vi "SingleOutPutA.vi"(8 "error in (no error)":errorcluster, 9 "Bool":bool, 10 "Index":i32, 11 "ZanCard in":refnum<class "ZanCard.lvclass">) -> (0 "error out":errorcluster, 3 "ZanCard out":refnum<class "ZanCard.lvclass">)   [LabVIEW 2019, in "ZanCard.lvclass"]
uses:
  ZanCard.lvclass
  ZanCard.lvclass/ZanCard.ctl
  LLB/zmotion/zaux/zauxdll.lvlib
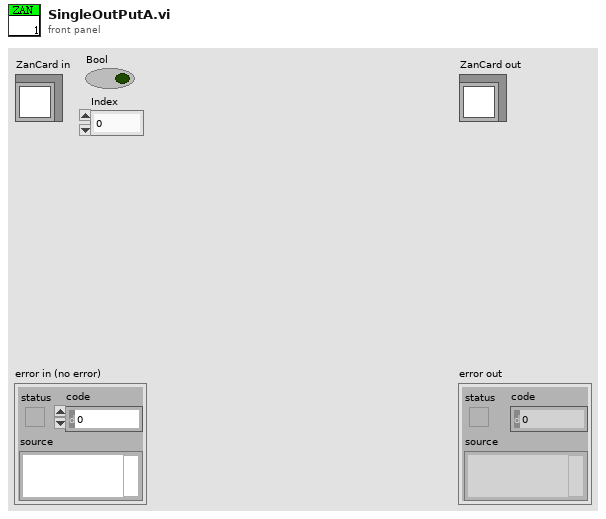
[diagram p1: front panel]
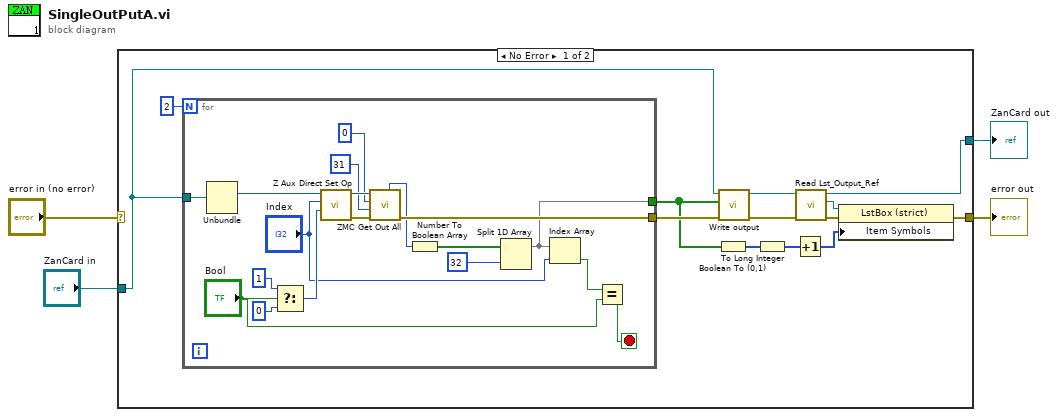
[diagram p0: block diagram]
diagram:
  n1 = case shown="No Error" "error in (no error)" {
    selector: "error in (no error)" -> [_ w37]
    tunnel: "ZanCard in" -> [w17 w36]
    tunnel: [w14 w36] -> w2
    tunnel: [w11 w37] -> w1
    frame No Error {
      n2 = for {
        N: 2 -> [_]
        tunnel: w17 -> [w31]
        tunnel: [w25] -> w10
        tunnel: [w19] -> w5
        stop <- w18 stop-if-true
        n3 = Unbundle(w31) -> (w35:i32)  [unwired: 3 out]
        n4 = Select(t=1, s="Bool", f=0) -> (s? t:f=w32:i32)
        n5 = call "Z Aux Direct Set Op.vi"("iValue"=w32, "ionum"="Index", "handle"=w35) -> ("error out"=w24:errorcluster, "handle out"=w30:u32)  [unwired: 6 in, 1 out]
        n6 = call "ZMC Get Out All.vi"("error in (no error)"=w24, "inumend"=31 ("ionumend"), "inumfirst"=0 ("ionumfirst"), "handle"=w30) -> ("error out"=w25:errorcluster, "pistate out"=w23:u32)  [unwired: 4 in, 2 out]
        n7 = Number To Boolean Array(number=w23) -> (Boolean array=w27:bool[])
        n8 = Split 1D Array(array=w27, index=32) -> (first subarray=w19:bool[])  [unwired: 1 out]
        n9 = Index Array(array=w19, index="Index") -> (element=w21:bool)
        n10 = Equal?(x=w21, y="Bool") -> (x = y?=w18:bool)
      }
      n11 = Boolean To (0,1)(Boolean=w5) -> (0, 1=w9:i16[])
      n12 = call-dynamic "Write output.vi"("error in (no error)"=w10, "output"=w5, "IOCard in"=w17) -> ("error out"=w13:errorcluster, "IOCard out"=w16:refnum<class "ZanCard.lvclass">)  [unwired: 7 in]
      n13 = To Long Integer(number=w9) -> (32bit integer=w8:i32[])
      n14 = Increment(x=w8) -> (x+1=w7:i32[])
      n15 = call-dynamic "Read Lst_Output_Ref.vi"("error in (no error)"=w13, "IOCard in"=w16) -> ("error out"=w12:errorcluster, "Lst_Output_Ref"=w15:refnum<vi>, "IOCard out"=w14:refnum<class "ZanCard.lvclass">)  [unwired: 7 in]
      n16 = property class="LstBox (strict)"(reference=w15, error in=w12, "Item Symbols"=w7) -> (error out=w11:errorcluster)  [unwired: 1 out]
    }
    frame Error {
    }
  }
  "error out" <- w1
  "ZanCard out" <- w2
